vi "Delete User.vi"(8 "error In":errorcluster) -> (0 "error Out":errorcluster)   [LabVIEW 2018]
uses:
  Control/Control 7.ctl
panel:
  in  "Selected User":string
  in  "Stop Button":bool
  in  "Login":bool
  in  "Enum":T1
  in  "Selection":string(combo)
  out "Login":bool
  in  "Password":string
  in  "User Name":string(combo)="VVDN TECH"
  in  "Delete User":bool
  in  "Project-Name":string="LensTuning"
  # "DELETE USERS"
  # "Admin Login"
  # "Delete User Details"
  # "Select User to Delete"
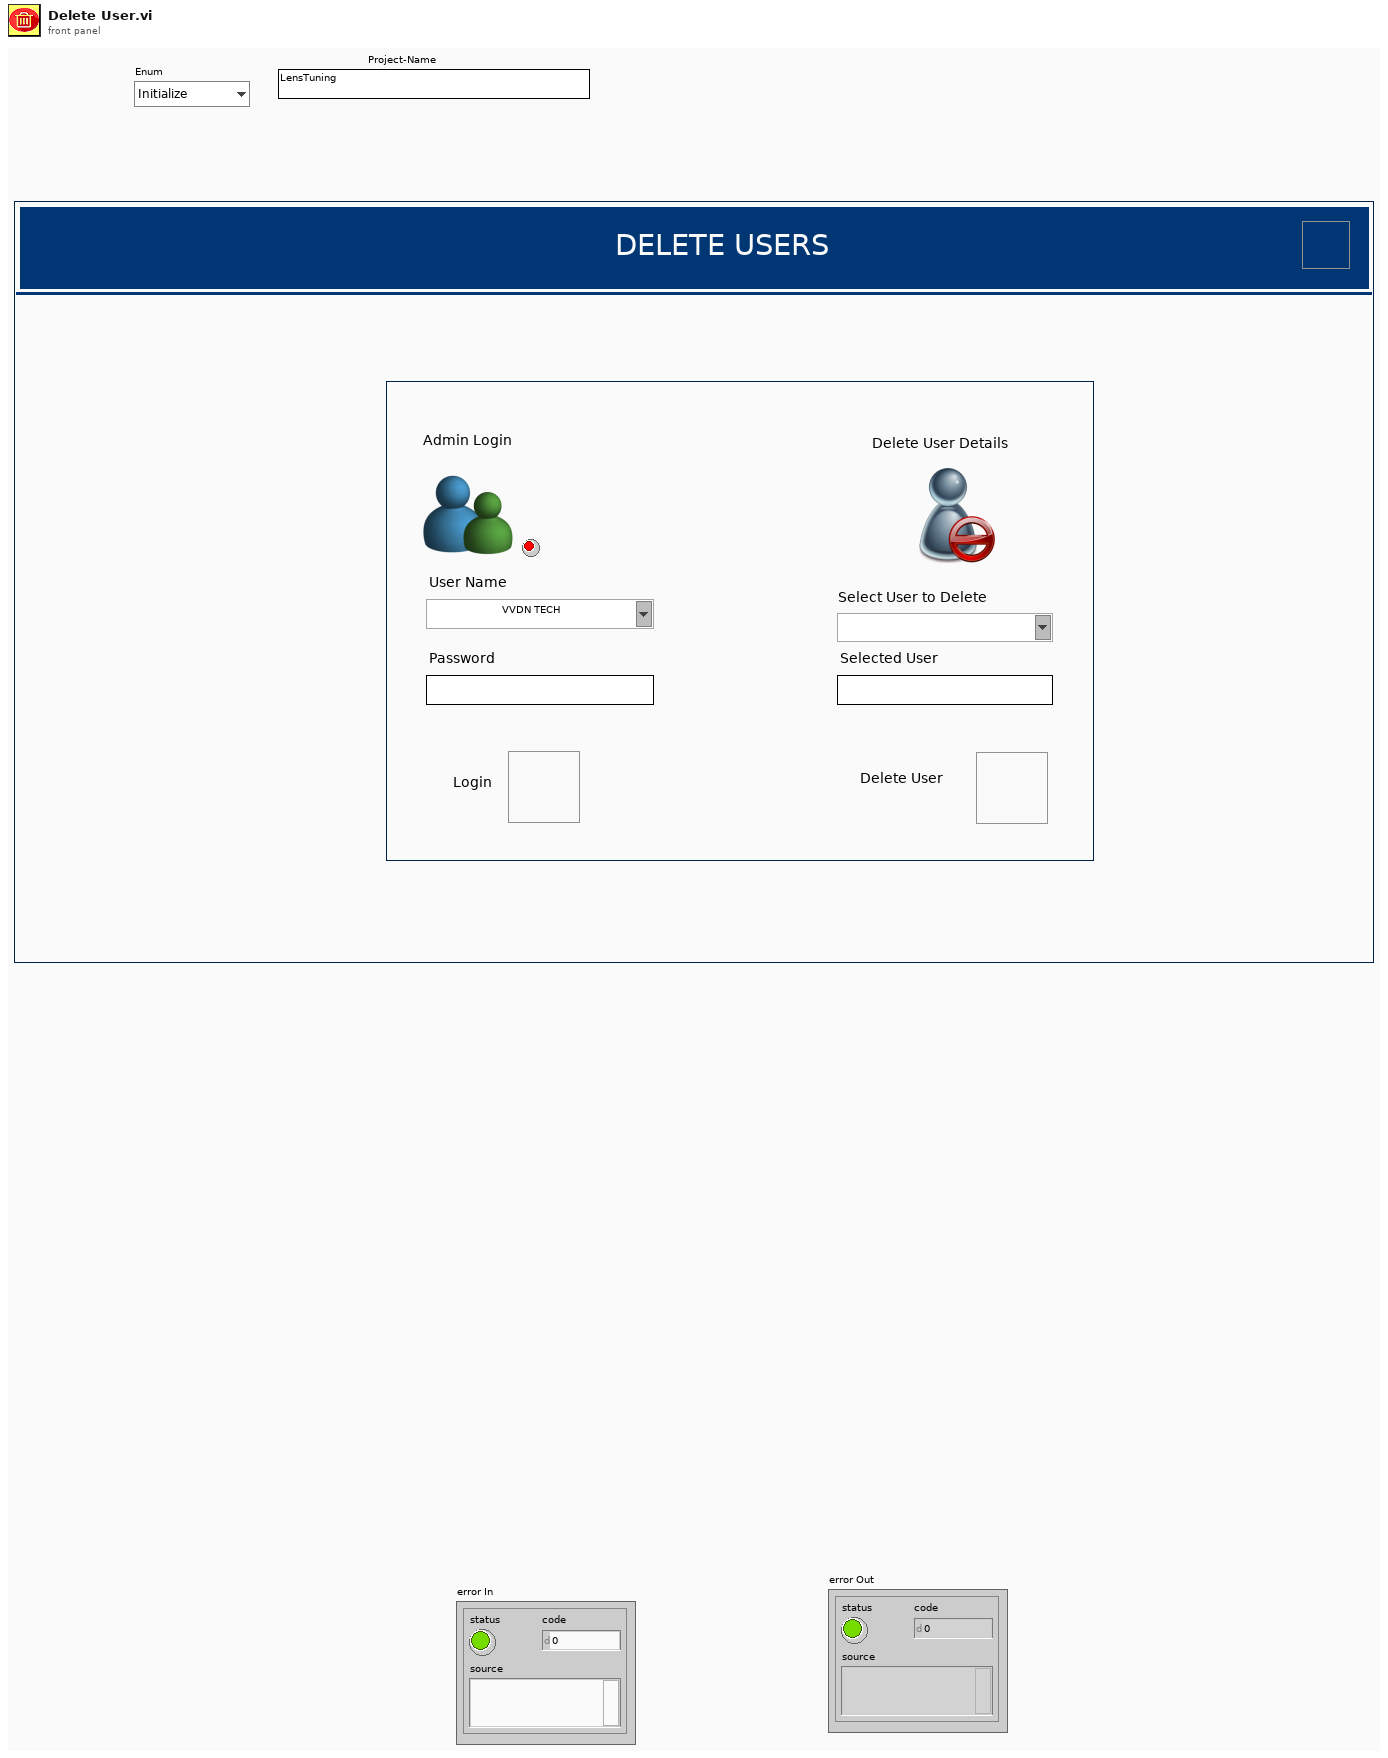
[diagram p1: front panel]
types:
  T1 = typedef "Control 7.ctl" = enum16{"Initialize", "Poll", "Login", "Add User", "Exit"}
  T2 = cluster{"Default User ":string, "Default Password":string, "Default User Type":u16}[]
  T3 = cluster{"Default User ":string, "Default Password":string, "Default User Type":u16}
  T4 = enum32{"Invalid", "Standard", "Closed", "Hidden", "Minimized", "Maximized"}
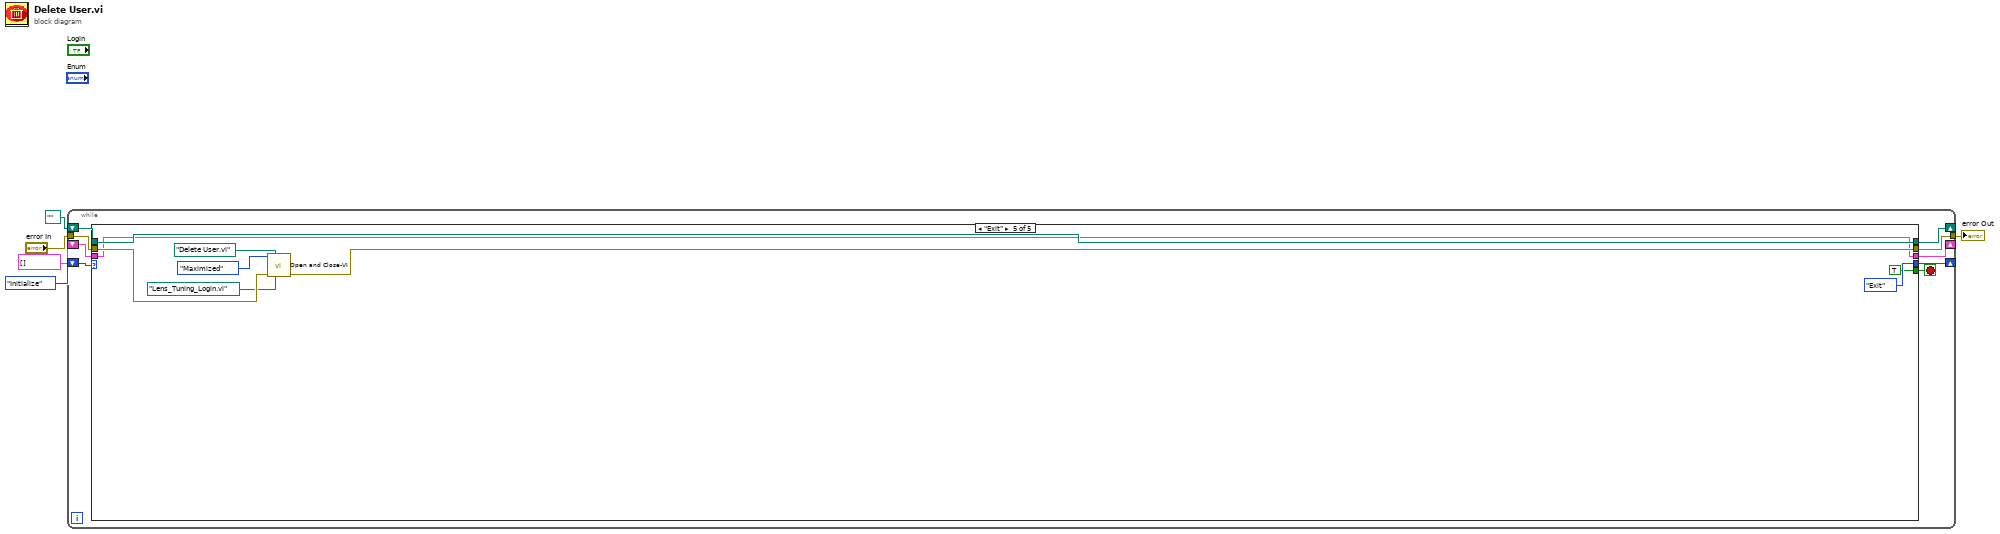
[diagram p0: block diagram]
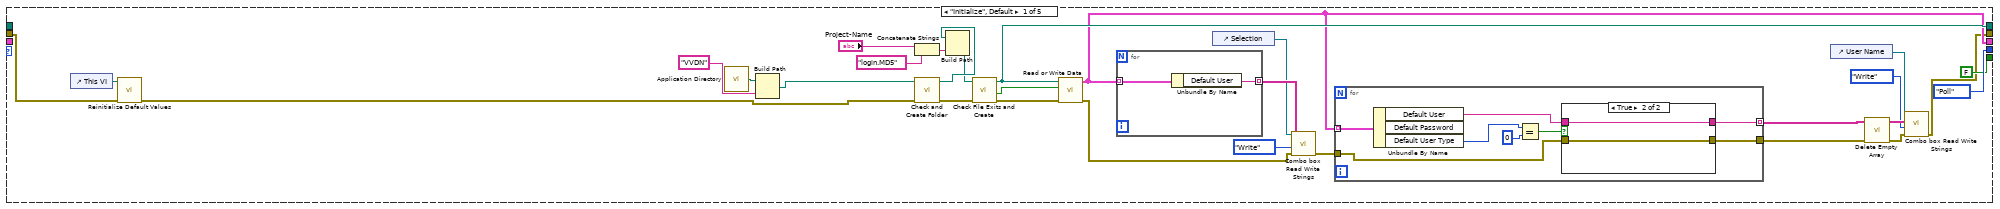
[diagram p2: hidden frame]
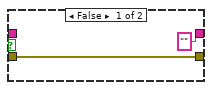
[diagram p3: hidden frame]
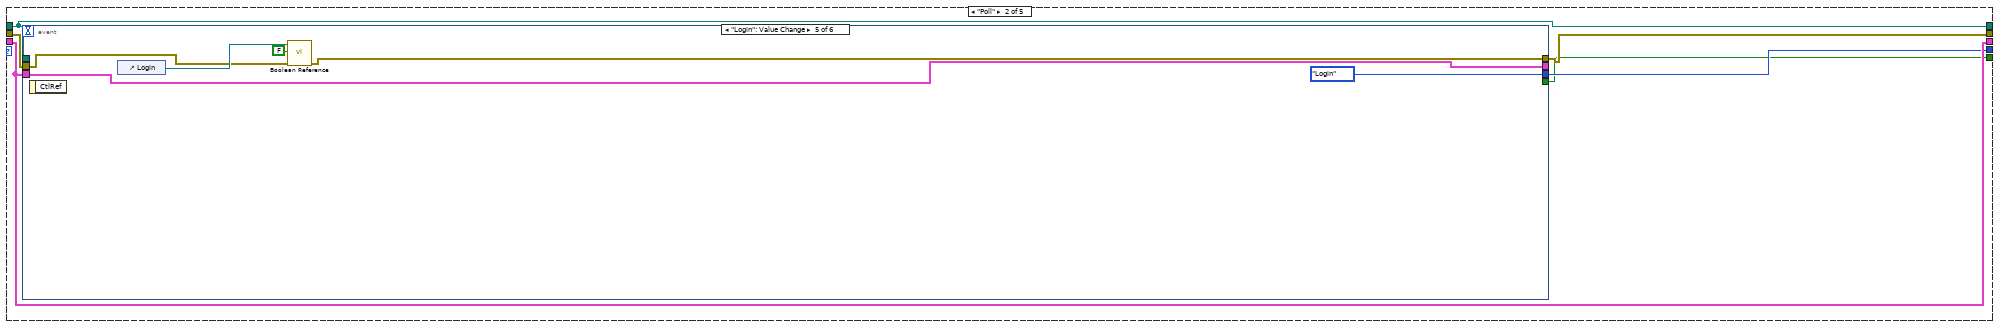
[diagram p4: hidden frame]
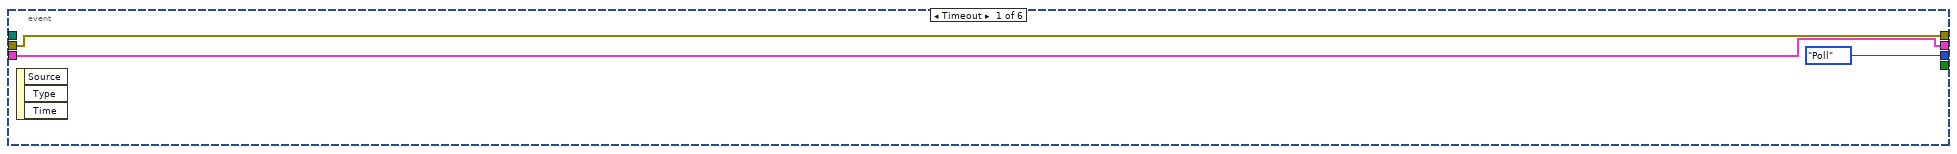
[diagram p5: hidden frame]
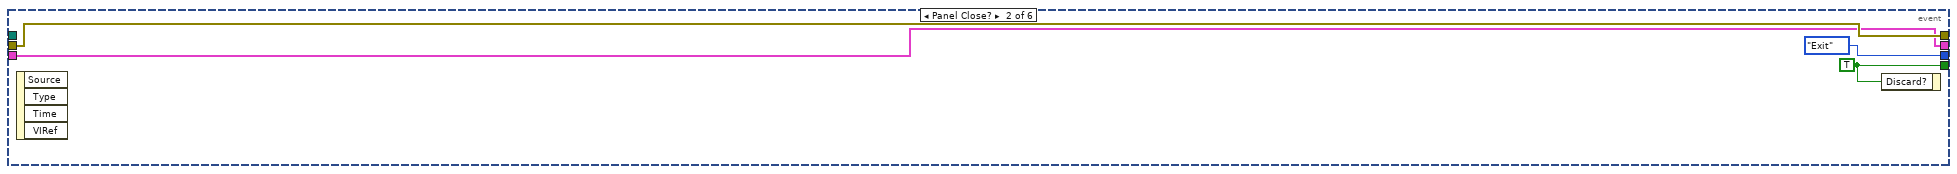
[diagram p6: hidden frame]
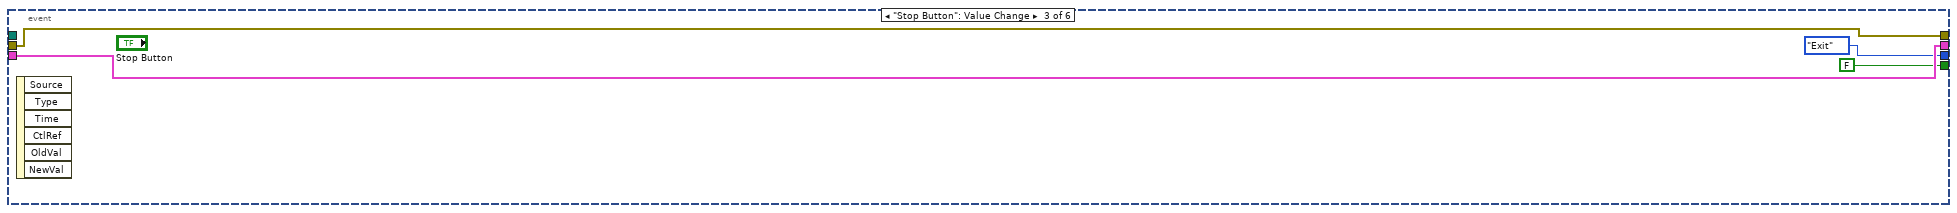
[diagram p7: hidden frame]
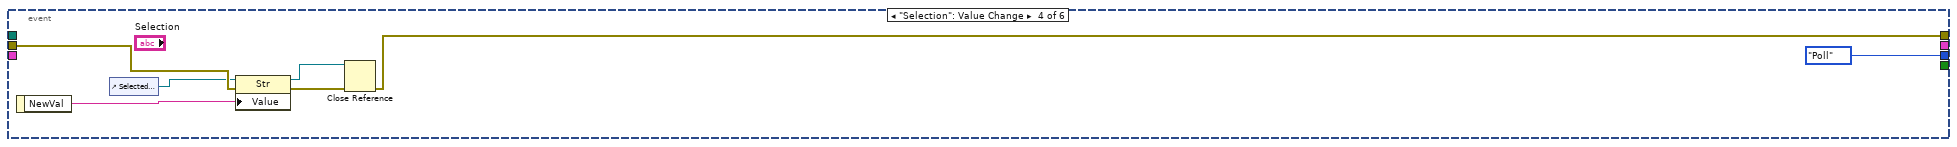
[diagram p8: hidden frame]
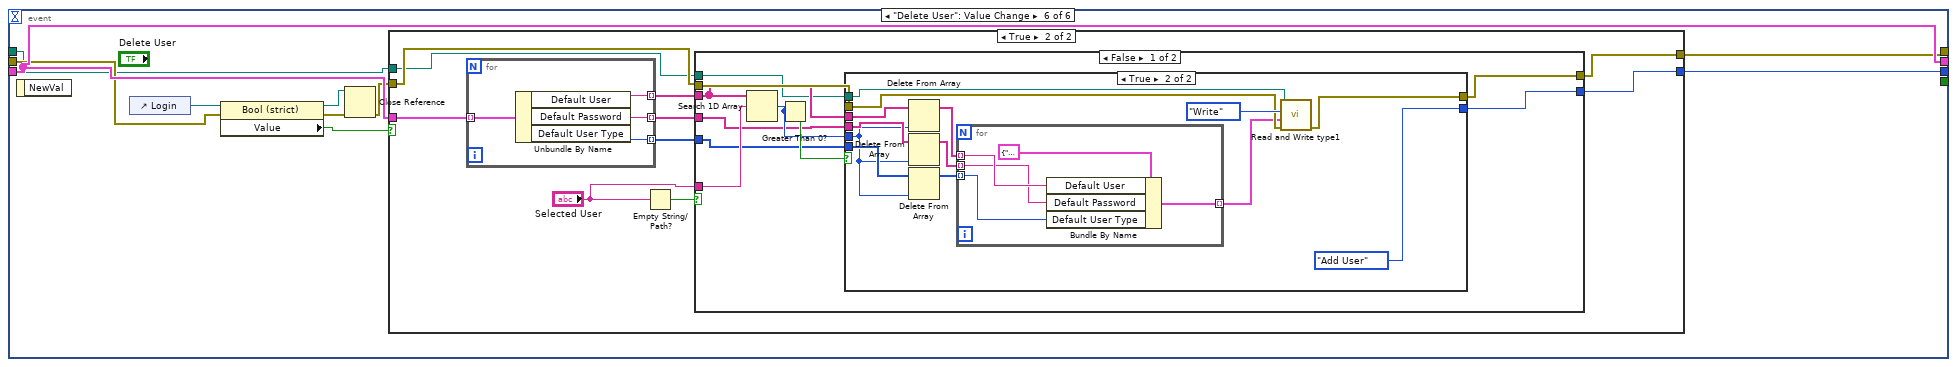
[diagram p9: hidden frame]
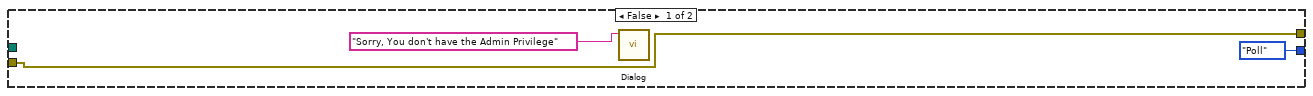
[diagram p10: hidden frame]
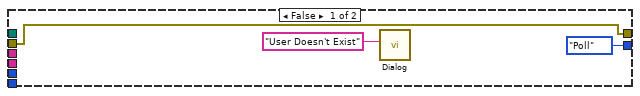
[diagram p11: hidden frame]
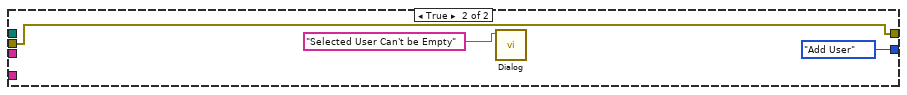
[diagram p12: hidden frame]
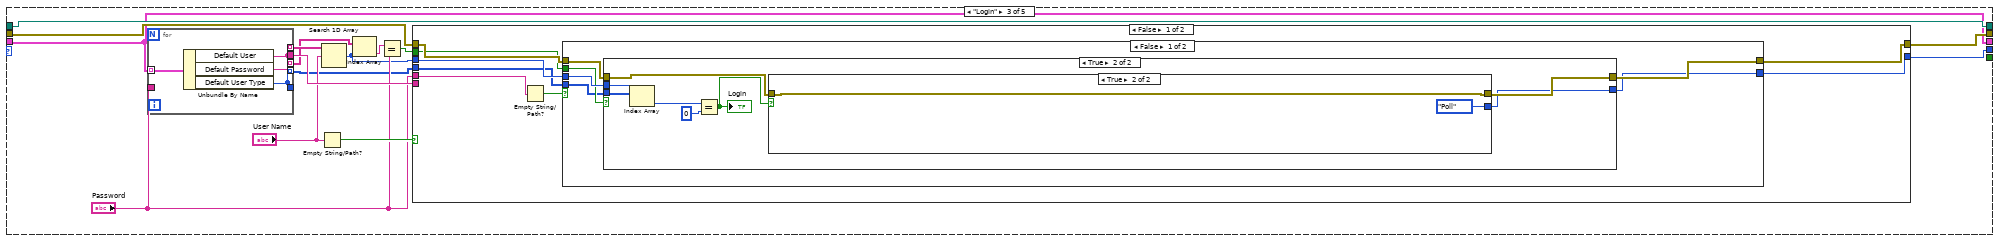
[diagram p13: hidden frame]
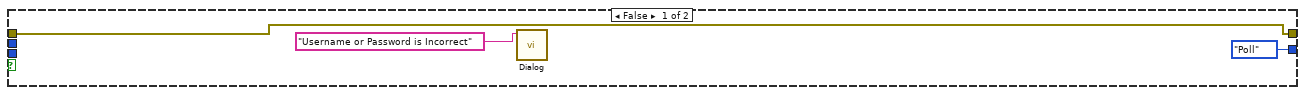
[diagram p14: hidden frame]
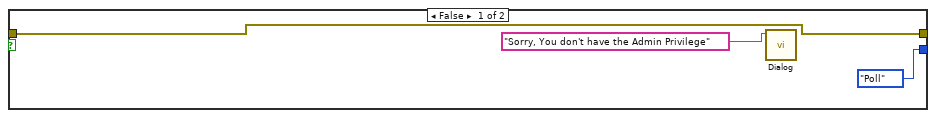
[diagram p15: hidden frame]
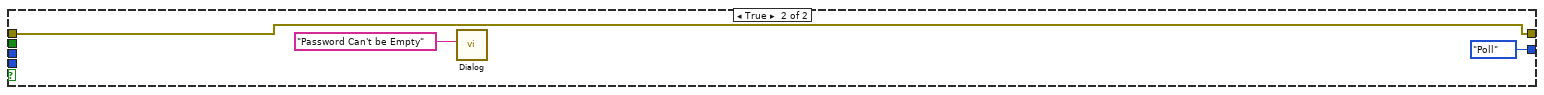
[diagram p16: hidden frame]
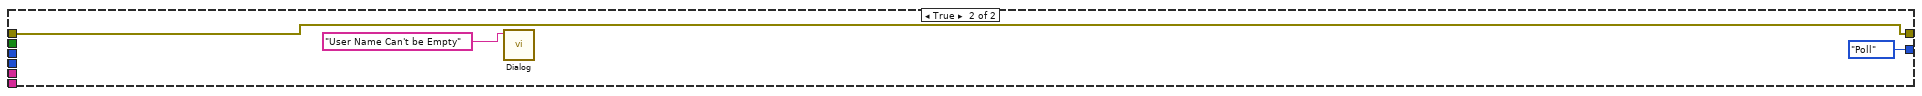
[diagram p17: hidden frame]
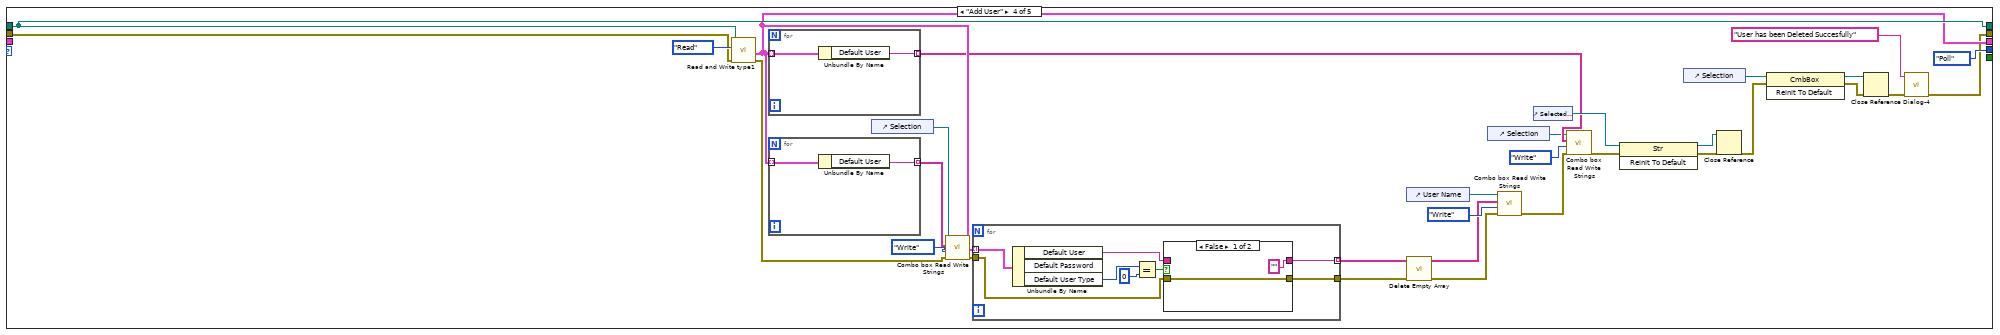
[diagram p18: hidden frame]
diagram:
  n1 = while {
    shift-right: [w10] -> _
    shift-left: Control_7."Initialize" ("Enum") -> [w14]
    tunnel: "error In" -> [w13]
    tunnel: [w12] -> w4
    shift-right: [w6] -> _
    shift-left: T2 [] ("User Details") -> [w11]
    shift-right: [w8] -> _
    shift-left: path "" ("Path Out") -> [w7]
    stop <- w9 stop-if-true
    n2 = case shown="\"Exit\"" w14 {
      tunnel: w13 -> [w27 w64 w164 w232 w259]
      tunnel: [w16 w62 w161 w219 w258] -> w12
      tunnel: w11 -> [_ w63 w158 _ w252]
      tunnel: [Control_7."Poll" ("Enum") w61 w162 Control_7."Poll" ("Enum") Control_7."Exit" ("Enum")] -> w10
      tunnel: [FALSE ("Discard?") w60 _ _ TRUE ("Discard?")] -> w9
      tunnel: [w31 w59 w159 w233 w253] -> w8
      tunnel: w7 -> [_ w59 w159 w233 w253]
      tunnel: [w28 w63 w158 w226 w252] -> w6
      frame "Initialize", Default {
        n3 = control-ref of="This VI"() -> (w25:refnum<vi>)
        n4 = call "Reinitialize Default Values.vi"("error in (no error)"=w27, "VI in"=w25) -> ("error out"=w26:errorcluster)  [unwired: 9 in]
        n5 = call <vilib>:"Application Directory.vi"() -> ("Application Directory"=w42:path)
        n6 = Build Path(base path=w42, name or relative path="VVDN") -> (appended path=w38:path)
        n7 = Concatenate Strings("Project-Name", "login.MD5" ("string")) -> (w36:string)
        n8 = call "Check and Create Folder.vi"("error in (no error)"=w26, "Path In"=w38) -> ("error out"=w35:errorcluster, "Path Out"=w37:path)  [unwired: 7 in, 1 out]
        n9 = Build Path(base path=w37, name or relative path=w36) -> (appended path=w34:path)
        n10 = call "Check File Exits and Create.vi"("error in"=w35, "Path In"=w34) -> ("error out"=w43:errorcluster, "file exists?"=w44:bool, "Path Out"=w31:path)  [unwired: 6 in, 1 out]
        n11 = call "Read or Write Data.vi"("error in"=w43, "file exists?"=w44, "Path Out"=w31) -> ("error out"=w22:errorcluster, "User Details"=w28:T2)  [unwired: 7 in]
        n12 = for {
          tunnel: w28 -> [w58] mode=indexing
          tunnel: [w57] -> w24 mode=indexing
          n13 = Unbundle By Name(w58) -> ("Default User"=w57:string)
        }
        n14 = control-ref of="Selection"() -> (w23:refnum<vi>)
        n15 = call "Combo box Read Write Strings.vi"("error in (no error)"=w22, "Enum"=enum16{"Read", "Write"}."Write", "Strings []"=w24, "ComboBox in"=w23) -> ("error out"=w21:errorcluster)  [unwired: 6 in, 1 out]
        n16 = for {
          tunnel: w28 -> [w52] mode=indexing
          tunnel: w21 -> [w47]
          tunnel: [w46] -> w30 mode=indexing
          tunnel: [w45] -> w29
          n17 = Unbundle By Name(w52) -> ("Default User"=w48:string, "Default User Type"=w51:u16)  [unwired: 1 out]
          n18 = Equal?(x=w51, y=u16 0) -> (x = y?=w49:bool)
          n19 = case shown="True" w49 {
            tunnel: w48 -> [_ w56]
            tunnel: ["" ("Default User") w56] -> w46
            tunnel: [w53 w55] -> w45
            tunnel: w47 -> [w53 w55]
            frame False {
            }
            frame True {
            }
          }
        }
        n20 = control-ref of="User Name"() -> (w19:refnum<vi>)
        n21 = call "Delete Empty Array.vi"("error in"=w29, "Array in"=w30) -> ("error out"=w18:errorcluster, "Array out"=w17:string[])  [unwired: 8 in]
        n22 = call "Combo box Read Write Strings.vi"("error in (no error)"=w18, "Enum"=enum16{"Read", "Write"}."Write", "Strings []"=w17, "ComboBox in"=w19) -> ("error out"=w16:errorcluster)  [unwired: 6 in, 1 out]
      }
      frame "Poll" {
        n23 = event shown="[4] \"Login\": Value Change" {
          selector: _ -> [_ _ _ _ _ _]
          dyn-events: _ -> [_ _ _ _ _ _]
          timeout: _ -> [_ _ _ _ _ _]
          tunnel: w64 -> [w65 w71 w73 w82 w84 w95]
          tunnel: w63 -> [w66 w70 w75 _ w88 w97]
          tunnel: [w66 w70 w75 _ w88 w97] -> _
          tunnel: [w65 w71 w73 w77 w83 w96] -> w62
          tunnel: [Control_7."Poll" ("Enum") Control_7."Exit" ("Enum") Control_7."Exit" ("Enum") Control_7."Poll" ("Enum") Control_7."Login" ("Enum") w98] -> w61
          tunnel: [_ w69 FALSE ("Discard?") _ _ _] -> w60
          tunnel: w59 -> [_ _ _ _ _ w89]
          event Timeout {
            n24 = event-data() -> ()  [unwired: 1 in, 3 out]
          }
          event Panel Close? {
            w69 = TRUE ("Discard?")
            n25 = event-data() -> ()  [unwired: 1 in, 4 out]
            n26 = event-data("Discard?"=w69) -> ()  [unwired: 1 in, 1 out]
          }
          event "Stop Button": Value Change {
            n27 = event-data() -> ()  [unwired: 1 in, 6 out]
          }
          event "Selection": Value Change {
            n28 = event-data() -> ("NewVal"=w80:string)  [unwired: 1 in]
            n29 = control-ref of="Selected User"() -> (w81:refnum<vi>)
            n30 = property class="Str"(reference=w81, error in=w82, "Value"=w80) -> (reference out=w79:refnum<vi>, error out=w78:errorcluster)
            n31 = Close Reference(reference=w79, error in (no error)=w78) -> (error out=w77:errorcluster)
          }
          event "Login": Value Change {
            n32 = event-data() -> ()  [unwired: 1 in, 1 out]
            n33 = control-ref of="Login"() -> (w86:refnum<vi>)
            n34 = call "Boolean Reference.vi"("error in"=w84, "Value"=FALSE, "Boolean in"=w86) -> ("error out"=w83:errorcluster)  [unwired: 8 in]
          }
          event "Delete User": Value Change {
            n35 = event-data() -> ()  [unwired: 1 in, 1 out]
            n36 = control-ref of="Login"() -> (w94:refnum<vi>)
            n37 = property class="Bool (strict)"(reference=w94, error in=w95) -> (reference out=w92:refnum<vi>, error out=w91:errorcluster, "Value"=w93:bool)
            n38 = Close Reference(reference=w92, error in (no error)=w91) -> (error out=w90:errorcluster)
            n39 = case shown="True" w93 {
              tunnel: [Control_7."Poll" ("Enum") w110] -> w98
              tunnel: w97 -> [_ w103]
              tunnel: w90 -> [w100 w108]
              tunnel: [w100 w107] -> w96
              tunnel: w89 -> [_ w102]
              frame False {
                n40 = call "Dialog.vi"("Status"="Sorry, You don't have the Admin Privilege") -> ()  [unwired: 10 in, 1 out]
              }
              frame True {
                n41 = for {
                  tunnel: w103 -> [w115] mode=indexing
                  tunnel: [w114] -> w109 mode=indexing
                  tunnel: [w113] -> w105 mode=indexing
                  tunnel: [w112] -> w104 mode=indexing
                  n42 = Unbundle By Name(w115) -> ("Default User"=w114:string, "Default Password"=w113:string, "Default User Type"=w112:u16)
                }
                n43 = Empty String/Path?(string/path="Selected User") -> (empty?=w111:bool)
                n44 = case shown="False" w111 {
                  tunnel: [w124 Control_7."Add User" ("Enum")] -> w110
                  tunnel: w109 -> [w120 _]
                  tunnel: w108 -> [w123 w147]
                  tunnel: [w122 w147] -> w107
                  tunnel: "Selected User" -> [w121 _]
                  tunnel: w105 -> [w118 _]
                  tunnel: w104 -> [w117 _]
                  tunnel: w102 -> [w116 _]
                  frame False {
                    n45 = Search 1D Array(1D array=w120, element=w121) -> (index of element=w119:i32)  [unwired: 1 in]
                    n46 = Greater Than 0?(x=w119) -> (x > 0?=w125:bool)
                    n47 = case shown="True" w125 {
                      tunnel: [Control_7."Poll" ("Enum") Control_7."Add User" ("Enum")] -> w124
                      tunnel: w123 -> [w128 w131]
                      tunnel: [w128 w130] -> w122
                      tunnel: w120 -> [_ w140]
                      tunnel: w119 -> [_ w137]
                      tunnel: w118 -> [_ w139]
                      tunnel: w117 -> [_ w138]
                      tunnel: w116 -> [_ w133]
                      frame False {
                        n48 = call "Dialog.vi"("Status"="User Doesn't Exist") -> ()  [unwired: 10 in, 1 out]
                      }
                      frame True {
                        n49 = Delete From Array(array=w140, index=w137) -> (array with subset deleted=w136:string[])  [unwired: 1 in, 1 out]
                        n50 = Delete From Array(array=w139, index=w137) -> (array with subset deleted=w135:string[])  [unwired: 1 in, 1 out]
                        n51 = Delete From Array(array=w138, index=w137) -> (array with subset deleted=w134:u16[])  [unwired: 1 in, 1 out]
                        n52 = for {
                          tunnel: w136 -> [w145] mode=indexing
                          tunnel: w135 -> [w144] mode=indexing
                          tunnel: w134 -> [w143] mode=indexing
                          tunnel: [w142] -> w129 mode=indexing
                          n53 = Bundle By Name(cluster=T3 {"Default User "="", "Default Password"="", "Default User Type"=0}, "Default User"=w145, "Default Password"=w144, "Default User Type"=w143) -> (w142:T3)
                        }
                        n54 = call "Read and Write type1.vi"("error in"=w131, "IN"=w129, "Enum"=enum16{"Init", "Read", "Write"}."Write", "Path Out"=w133) -> ("error out"=w130:errorcluster)  [unwired: 6 in, 1 out]
                      }
                    }
                  }
                  frame True {
                    n55 = call "Dialog.vi"("Status"="Selected User Can't be Empty") -> ()  [unwired: 10 in, 1 out]
                  }
                }
              }
            }
          }
        }
      }
      frame "Login" {
        n56 = for {
          tunnel: w158 -> [w168] mode=indexing
          tunnel: [w167] -> w160
          tunnel: "Password" -> [_]
          tunnel: [w165] -> _
          tunnel: [w167] -> w157 mode=indexing
          tunnel: [w166] -> w156 mode=indexing
          tunnel: [w165] -> w151 mode=indexing
          n57 = Unbundle By Name(w168) -> ("Default User"=w167:string, "Default Password"=w166:string, "Default User Type"=w165:u16)
        }
        n58 = Empty String/Path?(string/path="User Name") -> (empty?=w163:bool)
        n59 = Search 1D Array(1D array=w157, element="User Name") -> (index of element=w150:i32)  [unwired: 1 in]
        n60 = Index Array(array=w156, index=w150) -> (element=w155:string)
        n61 = Equal?(x=w155, y="Password") -> (x = y?=w153:bool)
        n62 = case shown="False" w163 {
          tunnel: w164 -> [w174 w202]
          tunnel: [w172 Control_7."Poll" ("Enum")] -> w162
          tunnel: [w173 w202] -> w161
          tunnel: w160 -> [_ _]
          tunnel: "Password" -> [w176 _]
          tunnel: w150 -> [w171 _]
          tunnel: w153 -> [w170 _]
          tunnel: w151 -> [w169 _]
          frame False {
            n63 = Empty String/Path?(string/path=w176) -> (empty?=w175:bool)
            n64 = case shown="False" w175 {
              tunnel: w174 -> [w182 w201]
              tunnel: [w181 w201] -> w173
              tunnel: [w180 Control_7."Poll" ("Enum")] -> w172
              tunnel: w171 -> [w179 _]
              tunnel: w170 -> [w178 _]
              tunnel: w169 -> [w177 _]
              frame False {
                n65 = case shown="True" w178 {
                  tunnel: w182 -> [w184 w192]
                  tunnel: [w184 w191] -> w181
                  tunnel: [Control_7."Poll" ("Enum") w190] -> w180
                  tunnel: w179 -> [_ w188]
                  tunnel: w177 -> [_ w187]
                  frame False {
                    n66 = call "Dialog.vi"("Status"="Username or Password is Incorrect") -> ()  [unwired: 10 in, 1 out]
                  }
                  frame True {
                    n67 = Index Array(array=w187, index=w188) -> (element=w186:u16)
                    n68 = Equal?(x=w186, y=u16 0) -> (x = y?=w189:bool)
                    "Login" <- w189
                    n69 = case shown="True" w189 {
                      tunnel: w192 -> [w195 w198]
                      tunnel: [w195 w198] -> w191
                      tunnel: [Control_7."Poll" ("Enum") Control_7."Poll" ("Enum")] -> w190
                      frame False {
                        n70 = call "Dialog.vi"("Status"="Sorry, You don't have the Admin Privilege") -> ()  [unwired: 10 in, 1 out]
                      }
                      frame True {
                      }
                    }
                  }
                }
              }
              frame True {
                n71 = call "Dialog.vi"("Status"="Password Can't be Empty") -> ()  [unwired: 10 in, 1 out]
              }
            }
          }
          frame True {
            n72 = call "Dialog.vi"("Status"="User Name Can't be Empty") -> ()  [unwired: 10 in, 1 out]
          }
        }
      }
      frame "Add User" {
        n73 = call "Read and Write type1.vi"("error in"=w232, "Enum"=enum16{"Init", "Read", "Write"}."Read", "Path Out"=w233) -> ("error out"=w216:errorcluster, "OUT"=w226:T2)  [unwired: 7 in]
        n74 = for {
          tunnel: w226 -> [w237] mode=indexing
          tunnel: [w236] -> w207 mode=indexing
          n75 = Unbundle By Name(w237) -> ("Default User"=w236:string)
        }
        n76 = for {
          tunnel: w226 -> [w251] mode=indexing
          tunnel: [w250] -> w215 mode=indexing
          n77 = Unbundle By Name(w251) -> ("Default User"=w250:string)
        }
        n78 = control-ref of="Selection"() -> (w217:refnum<vi>)
        n79 = call "Combo box Read Write Strings.vi"("error in (no error)"=w216, "Enum"=enum16{"Read", "Write"}."Write", "Strings []"=w215, "ComboBox in"=w217) -> ("error out"=w214:errorcluster)  [unwired: 6 in, 1 out]
        n80 = for {
          tunnel: w226 -> [w245] mode=indexing
          tunnel: w214 -> [w240]
          tunnel: [w239] -> w231 mode=indexing
          tunnel: [w238] -> w230
          n81 = Unbundle By Name(w245) -> ("Default User"=w241:string, "Default User Type"=w244:u16)  [unwired: 1 out]
          n82 = Equal?(x=w244, y=u16 0) -> (x = y?=w242:bool)
          n83 = case shown="False" w242 {
            tunnel: w241 -> [_ w249]
            tunnel: ["" ("Default User") w249] -> w239
            tunnel: [w246 w248] -> w238
            tunnel: w240 -> [w246 w248]
            frame False {
            }
            frame True {
            }
          }
        }
        n84 = control-ref of="User Name"() -> (w212:refnum<vi>)
        n85 = call "Delete Empty Array.vi"("error in"=w230, "Array in"=w231) -> ("error out"=w210:errorcluster, "Array out"=w211:string[])  [unwired: 8 in]
        n86 = control-ref of="Selection"() -> (w206:refnum<vi>)
        n87 = call "Combo box Read Write Strings.vi"("error in (no error)"=w210, "Enum"=enum16{"Read", "Write"}."Write", "Strings []"=w211, "ComboBox in"=w212) -> ("error out"=w208:errorcluster)  [unwired: 6 in, 1 out]
        n88 = control-ref of="Selected User"() -> (w229:refnum<vi>)
        n89 = call "Combo box Read Write Strings.vi"("error in (no error)"=w208, "Enum"=enum16{"Read", "Write"}."Write", "Strings []"=w207, "ComboBox in"=w206) -> ("error out"=w205:errorcluster)  [unwired: 6 in, 1 out]
        n90 = invoke class="Str" method="Reinit To Default"(reference=w229, error in=w205) -> (reference out=w228:refnum<vi>, error out=w227:errorcluster)  [unwired: 1 in, 1 out]
        n91 = control-ref of="Selection"() -> (w225:refnum<vi>)
        n92 = Close Reference(reference=w228, error in (no error)=w227) -> (error out=w222:errorcluster)
        n93 = invoke class="CmbBox" method="Reinit To Default"(reference=w225, error in=w222) -> (reference out=w224:refnum<vi>, error out=w223:errorcluster)  [unwired: 1 in, 1 out]
        n94 = Close Reference(reference=w224, error in (no error)=w223) -> (error out=w220:errorcluster)
        n95 = call "Dialog-4.vi"("error in"=w220, "Status"="User has been Deleted Succesfully") -> ("error out"=w219:errorcluster)  [unwired: 8 in, 1 out]
      }
      frame "Exit" {
        n96 = call "Open and Close-VI.vi"("State"=T4."Maximized", "Close VI"=path "Delete User.vi", "error in"=w259, "Open VI"=path "Lens_Tuning_Login.vi") -> ("error out"=w258:errorcluster)  [unwired: 11 in]
      }
    }
  }
  "error Out" <- w4
